vi "InterfaceSelect.vi"(8 "error in (no error)":errorcluster, 10 "Interface Select BOX":enum32{"Gigabit Ethernet", "IEEE1394", "PCI"}(radio)) -> (0 "error out":errorcluster, 1 "Out_IP Address":T1 caption="Info_IP Address" {"Manual_IP"."IP4" format="%.03d"; "Manual_IP"."IP3" format="%.03d"; "Manual_IP"."IP2" format="%.03d"; "Manual_IP"."IP1" format="%.03d"; "Auto_IP"."IP3" format="%.03d"; "Auto_IP"."IP2" format="%.03d"; "Auto_IP"."IP1" format="%.03d"}, 2 "nInterfaceCode":u32 format="%.0x")   [LabVIEW 2015]
panel:
  in  "IP Address":T1 {"Manual_IP"."IP4" format="%.03d"; "Manual_IP"."IP3" format="%.03d"; "Manual_IP"."IP2" format="%.03d"; "Manual_IP"."IP1" format="%.03d"; "Auto_IP"."IP3" format="%.03d"; "Auto_IP"."IP2" format="%.03d"; "Auto_IP"."IP1" format="%.03d"}
  in  "OK_Btn":bool
  # "．"
  # "．"
  # "．"
  # "．"
  # "．"
  # "．"
  # "XXX"
  # "."
  # "."
  # "."
  # "."
  # "."
  # "."
  # "XXX"
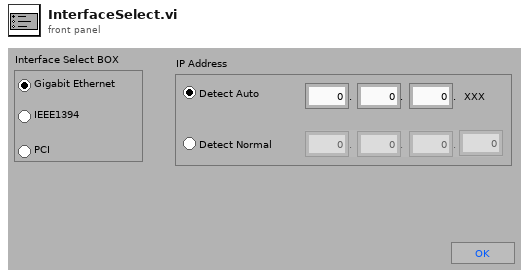
[diagram p1: front panel]
types:
  T1 = cluster{"Detect Select BOX":enum32{"Detect Auto", "Detect Normal"}, "Auto_IP":cluster{"IP1":u8, "IP2":u8, "IP3":u8}, "Manual_IP":cluster{"IP1":u8, "IP2":u8, "IP3":u8, "IP4":u8}}
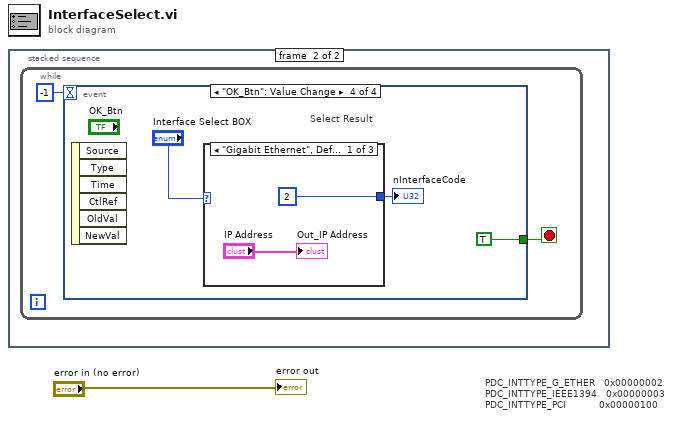
[diagram p0: block diagram]
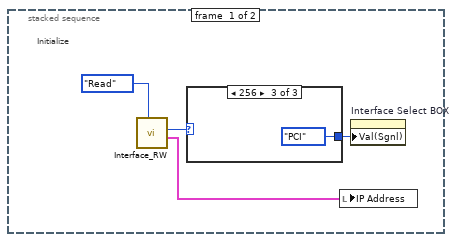
[diagram p2: hidden frame]
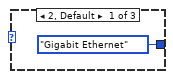
[diagram p3: hidden frame]
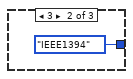
[diagram p4: hidden frame]
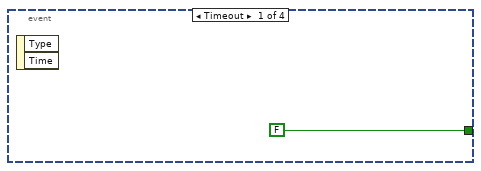
[diagram p5: hidden frame]
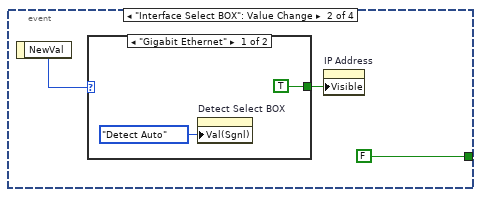
[diagram p6: hidden frame]
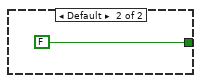
[diagram p7: hidden frame]
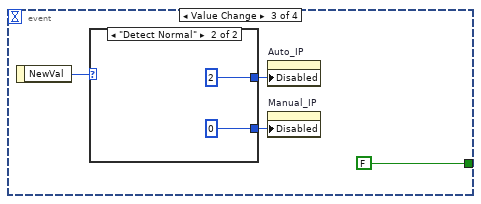
[diagram p8: hidden frame]
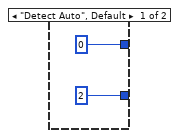
[diagram p9: hidden frame]
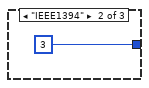
[diagram p10: hidden frame]
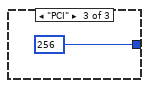
[diagram p11: hidden frame]
diagram:
  # "PDC_INTTYPE_G_ETHER\t\t\t0x00000002\nPDC_INTTYPE_IEEE1394\t\t\t0x00000003\nPDC_INTTYPE_PCI\t\t\t\t\t\t     0x00000100"
  n1 = stacked-sequence {
    frame #0 {
      # "Initialize"
      n2 = call "Interface_RW.vi"("Mode"=enum16{"Write", "Read"}."Read") -> ("Out_IP Address"=w2:T1, "Out_InterfaceCode"=w3:u32)  [unwired: 3 in, 6 out]
      n3 = case shown="256" w3 {
        tunnel: [enum32{"Gigabit Ethernet", "IEEE1394", "PCI"}."Gigabit Ethernet" ("値 (信号)") enum32{"Gigabit Ethernet", "IEEE1394", "PCI"}."IEEE1394" ("値 (信号)") enum32{"Gigabit Ethernet", "IEEE1394", "PCI"}."PCI" ("値 (信号)")] -> w5
        frame 2, Default {
        }
        frame 3 {
        }
        frame 256 {
        }
      }
      n4 = local write "IP Address"(w2) -> ()
      n5 = property on="Interface Select BOX" class="RadioBtnsControl (strict)"("Val(Sgnl)"=w5) -> ()  [unwired: 2 in, 2 out]
    }
    frame #1 {
      n6 = while {
        stop <- w9 stop-if-true
        n7 = event shown="[3] \"OK_Btn\": Value Change" {
          selector: _ -> [_ _ _ _]
          dyn-events: _ -> [_ _ _ _]
          timeout: -1 -> [_ _ _ _]
          tunnel: [FALSE FALSE FALSE TRUE] -> w9
          event Timeout {
            n8 = event-data() -> ()  [unwired: 3 out]
          }
          event "Interface Select BOX": Value Change {
            n9 = event-data() -> ("NewVal"=w14:enum32{"Gigabit Ethernet", "IEEE1394", "PCI"})  [unwired: 1 out]
            n10 = case shown="\"Gigabit Ethernet\"" w14 {
              tunnel: [TRUE FALSE] -> w13
              frame "Gigabit Ethernet" {
                n11 = property on="Detect Select BOX" class="RadioBtnsControl (strict)"("Val(Sgnl)"=enum32{"Detect Auto", "Detect Normal"}."Detect Auto" ("値 (信号)")) -> ()  [unwired: 2 in, 2 out]
              }
              frame Default {
              }
            }
            n12 = property on="IP Address" class="Clust (strict)"("Visible"=w13) -> ()  [unwired: 2 in, 2 out]
          }
          event "IP Address.Detect Select BOX": Value Change {
            n13 = event-data() -> ("NewVal"=w21:enum32{"Detect Auto", "Detect Normal"})  [unwired: 1 out]
            n14 = case shown="\"Detect Normal\"" w21 {
              tunnel: [u8 0 ("無効") u8 2 ("無効")] -> w20
              tunnel: [u8 2 ("無効") u8 0 ("無効")] -> w19
              frame "Detect Auto", Default {
              }
              frame "Detect Normal" {
              }
            }
            n15 = property on="Auto_IP" class="Clust (strict)"("Disabled"=w20) -> ()  [unwired: 2 in, 2 out]
            n16 = property on="Manual_IP" class="Clust (strict)"("Disabled"=w19) -> ()  [unwired: 2 in, 2 out]
          }
          event "OK_Btn": Value Change {
            # "Select Result"
            n17 = event-data() -> ()  [unwired: 7 out]
            n18 = case shown="\"Gigabit Ethernet\", Default" "Interface Select BOX" {
              tunnel: [u32 2 u32 3 u32 256] -> w26
              frame "Gigabit Ethernet", Default {
                "Out_IP Address" <- "IP Address"
              }
              frame "IEEE1394" {
              }
              frame "PCI" {
              }
            }
            "nInterfaceCode" <- w26
          }
        }
      }
    }
  }
  "error out" <- "error in (no error)"
